vi "Create User Event - Stop.vi"(8 "entrée d'erreur (pas d'erreur)":errorcluster) -> (0 "sortie d'erreur":errorcluster, 2 "Événement utilisateur - Arrêt":refnum<user-event>, 3 "Refnum Enregistrement à l'événement Arrêt":refnum<event-registration>)   [LabVIEW 2016, in "User Event - Stop.lvlib"]
doc: "Créer un événement utilisateur booléen qui sera utilisé pour arrêter la boucle d'événement à partir de la boucle de gestion de messages."
uses:
  User Event - Stop.lvlib
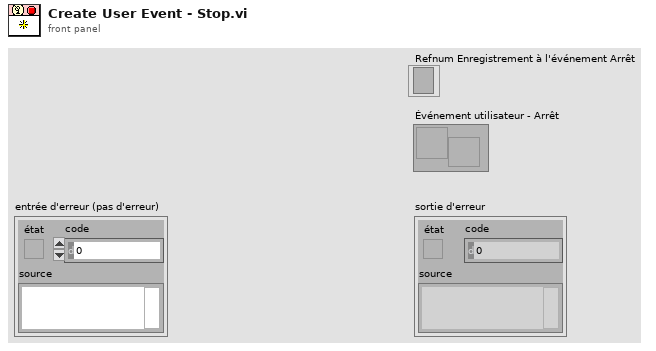
[diagram p1: front panel]
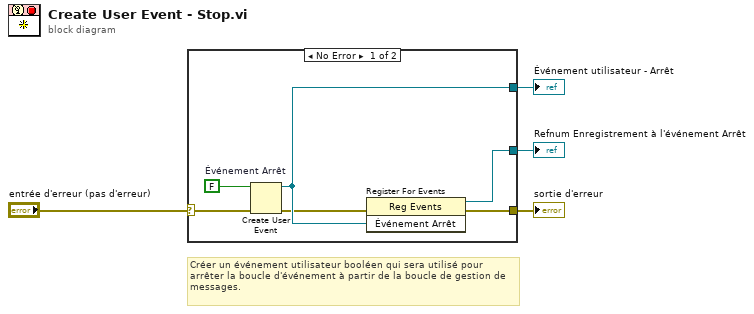
[diagram p0: block diagram]
diagram:
  # "Créer un événement utilisateur booléen qui sera utilisé pour arrêter la boucle d'événement à partir de la boucle de gestion de messages."
  n1 = case shown="No Error" "entrée d'erreur (pas d'erreur)" {
    selector: "entrée d'erreur (pas d'erreur)" -> [w5 w11]
    tunnel: [w10 _] -> w4
    tunnel: [w9 _] -> w3
    tunnel: [w6 w11] -> w2
    frame No Error {
      w8 = FALSE  # Événement Arrêt
      n2 = Create User Event(user event datatype=w8, error in=w5) -> (user event=w10:refnum<user-event>, error out=w7:errorcluster)
      n3 = register-events(error in=w7, w10) -> (reference out=w9:refnum<event-registration>, error out=w6:errorcluster)  [unwired: 1 in]
    }
    frame Error {
    }
  }
  "Événement utilisateur - Arrêt" <- w4
  "sortie d'erreur" <- w2
  "Refnum Enregistrement à l'événement Arrêt" <- w3
